vi "CreatePrivateEvents.vi"(8 "error in (no error)":errorcluster, 11 "Lockin.DAQ":refnum<class "Instrument.DAQ.lvclass">) -> (0 "error out":errorcluster, 3 "Lockin.DAQ out":refnum<class "Instrument.DAQ.lvclass">)   [LabVIEW 2019, in "Instrument.Lockin.lvlib" / "Instrument.DAQ.lvclass"]
doc: "---------------------------------------------------------------\nJKI State Machine Objects™\nhttp://jki.net/state-machine-objects/\nCopyright (C) 2005-2015, JKI <info@jki.net>\nALL RIGHTS RESERVEDJKI State Machine Objects (SMO) 1.0.0.4\nJKI - JKI\nCopyright (c) 2015, JKI"
uses:
  Instrument.DAQ.lvclass
  Typedefs/PrivateEvents--DAQ.setAOconfig.ctl
  Typedefs/DAQ.Config.AO--Cluster--Array.ctl
  Typedefs/DAQ.Config.AO.Range--enum.ctl
  Typedefs/DAQ.TerminalConfiguration--ring.ctl
  Typedefs/DAQ.Type--enum.ctl
  Typedefs/PrivateEvents--DAQ.setAIconfig.ctl
  Typedefs/DAQ.Config.AI--Cluster--Array.ctl
  Typedefs/DAQ.Config.AI.Coupling--enum.ctl
  Typedefs/DAQ.Config.AI.Range--enum.ctl
  DAQmx/typedefs/Simulation Mode--enum.ctl
  Typedefs/PrivateEvents--DAQ.setAO.ctl
  Typedefs/AO.Channel--Cluster--Array.ctl
  Typedefs/AO.Channel--Cluster.ctl
  Typedefs/AO.Channel.Function--Enum.ctl
  Typedefs/PrivateEvents--DAQ.setREF.ctl
  Typedefs/REF.Channel--Cluster--Array.ctl
  Typedefs/REF.Channel--Cluster.ctl
  Typedefs/PrivateEvents--DAQ.setSampling.ctl
  Typedefs/DAQ.Sampling--Cluster.ctl
  Typedefs/DAQ.Sampling.Sampling--Cluster.ctl
  Typedefs/PrivateEvents--DAQ.setState.ctl
  Typedefs/State--enum.ctl
  Typedefs/PrivateEvents--DAQ.setInputGain.ctl
  Typedefs/PrivateEvents--DAQ.setSweep.ctl
  Typedefs/Sweep.Configuration--Cluster.ctl
  Typedefs/Sweep.Channel--Cluster--Array.ctl
  Typedefs/Sweep.Channel--Cluster.ctl
  Typedefs/Sweep.Pattern--Enum.ctl
  Typedefs/PrivateEvents--DAQ.measureOffset.ctl
  Typedefs/PrivateEvents--DAQ.zeroOffset.ctl
  Typedefs/PrivateEvents--DAQ.setPreFilter.ctl
  Typedefs/Configuration.Prefilter--Cluster.ctl
  Typedefs/PrivateEvents--DAQ.autoConfigureDAQ.ctl
  Typedefs/PrivateEvents--DAQ.setCalibration.ctl
  Typedefs/PrivateEvents--DAQ.setOutputGain.ctl
  Typedefs/PrivateEvents--DAQ.setAI.ctl
  Typedefs/AI.Channel--Cluster--Array.ctl
  Typedefs/AI.Channel--Cluster.ctl
  Typedefs/PrivateEvents--DAQ.zeroPhase.ctl
  Typedefs/PrivateEvents--DAQ.setAmplitudeLimit.ctl
  Typedefs/Configuration.AmplitudeLimit--Cluster.ctl
  Typedefs/PrivateEvents--DAQ.setLinkFrequencies.ctl
  Typedefs/Configuration.LinkFrequencies--Cluster.ctl
  Typedefs/PrivateEvents--DAQ.showUI.ctl
  Typedefs/PrivateEvents--DAQ.setInputOffset.ctl
  Typedefs/PrivateEvents--DAQ.setDCLimit.ctl
  Typedefs/Configuration.DCLimit--Cluster.ctl
  Typedefs/PrivateEvents--DAQ.setDutyCycle.ctl
  Typedefs/Configuration.DutyCycle--Cluster.ctl
  Instrument.DAQ.lvclass/Instrument.DAQ.ctl
  <vilib>/JKI/JKI SMO/SMO/SMO.lvclass
  DAQmx/DAQmx.lvclass
panel:
  # "For instructions on how to use the JKI State Machine Objects, examples and video tutorials, visit:\nhttp://jki.net/state-machine-objects/\n\nJKI State Machine Objects™\nhttp://jki.net/state-machine-objects/\nCopyright (C) 2005-2015, JKI <info@jki.net>\nALL RIGHTS RESERVED"
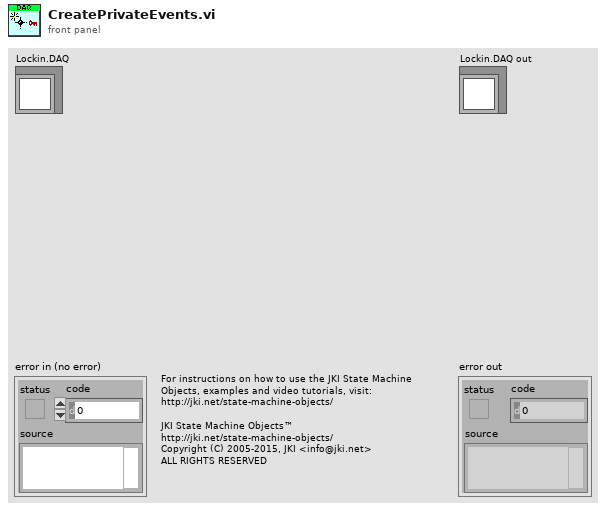
[diagram p1: front panel]
types:
  T1 = typedef "Instrument.Lockin.lvlib/Instrument.DAQ.lvclass/PrivateEvents--DAQ.setDutyCycle.ctl" = cluster{"Duty Cycle":T2}
  T2 = typedef "Instrument.Lockin.lvlib/Instrument.DAQ.lvclass/Configuration.DutyCycle--Cluster.ctl" = cluster{"Option?":bool, "Duty Cycle (%)":dbl}
  T3 = typedef "Instrument.Lockin.lvlib/Instrument.DAQ.lvclass/PrivateEvents--DAQ.setDCLimit.ctl" = cluster{"DC Limit":T4}
  T4 = typedef "Instrument.Lockin.lvlib/Instrument.DAQ.lvclass/Configuration.DCLimit--Cluster.ctl" = cluster{"Limit (V)":dbl}
  T5 = typedef "Instrument.Lockin.lvlib/Instrument.DAQ.lvclass/PrivateEvents--DAQ.setInputOffset.ctl" = cluster{"Input Offset":dbl[]}
  T6 = typedef "Instrument.Lockin.lvlib/Instrument.DAQ.lvclass/PrivateEvents--DAQ.showUI.ctl" = bool
  T7 = typedef "Instrument.Lockin.lvlib/Instrument.DAQ.lvclass/PrivateEvents--DAQ.setLinkFrequencies.ctl" = cluster{"Link Frequencies":T8}
  T8 = typedef "Instrument.Lockin.lvlib/Instrument.DAQ.lvclass/Configuration.LinkFrequencies--Cluster.ctl" = cluster{"Link?":bool, "Frequency (Hz)":dbl}
  T9 = typedef "Instrument.Lockin.lvlib/Instrument.DAQ.lvclass/PrivateEvents--DAQ.setAmplitudeLimit.ctl" = cluster{"Amplitude Limit ":T10}
  T10 = typedef "Instrument.Lockin.lvlib/Instrument.DAQ.lvclass/Configuration.AmplitudeLimit--Cluster.ctl" = cluster{"Limit (V)":dbl}
  T11 = typedef "Instrument.Lockin.lvlib/Instrument.DAQ.lvclass/PrivateEvents--DAQ.zeroPhase.ctl" = bool
  T12 = typedef "Instrument.Lockin.lvlib/Instrument.DAQ.lvclass/PrivateEvents--DAQ.setAI.ctl" = cluster{"AI Channels":T13}
  T13 = typedef "Instrument.Lockin.lvlib/Instrument.DAQ.lvclass/AI.Channel--Cluster--Array.ctl" = T14[]
  T14 = typedef "Instrument.Lockin.lvlib/Instrument.DAQ.lvclass/AI.Channel--Cluster.ctl" = cluster{"Enable?":bool, "Channel":i32, "References":u16[], "reference index":i32}
  T15 = typedef "Instrument.Lockin.lvlib/Instrument.DAQ.lvclass/PrivateEvents--DAQ.setOutputGain.ctl" = cluster{"Output Gain":dbl[]}
  T16 = typedef "Instrument.Lockin.lvlib/Instrument.DAQ.lvclass/PrivateEvents--DAQ.setCalibration.ctl" = enum16{"Check", "Calibrate"}
  T17 = typedef "Instrument.Lockin.lvlib/Instrument.DAQ.lvclass/PrivateEvents--DAQ.autoConfigureDAQ.ctl" = bool
  T18 = typedef "Instrument.Lockin.lvlib/Instrument.DAQ.lvclass/PrivateEvents--DAQ.setPreFilter.ctl" = cluster{"PreFilter":T19}
  T19 = typedef "Instrument.Lockin.lvlib/Instrument.DAQ.lvclass/Configuration.Prefilter--Cluster.ctl" = cluster{"60 Hz":bool, "Low Pass":bool, "Low Pass Cutoff (Hz)":dbl}
  T20 = typedef "Instrument.Lockin.lvlib/Instrument.DAQ.lvclass/PrivateEvents--DAQ.zeroOffset.ctl" = bool
  T21 = typedef "Instrument.Lockin.lvlib/Instrument.DAQ.lvclass/PrivateEvents--DAQ.measureOffset.ctl" = bool
  T22 = typedef "Instrument.Lockin.lvlib/Instrument.DAQ.lvclass/PrivateEvents--DAQ.setSweep.ctl" = cluster{"setSweep":T23}
  T23 = typedef "Instrument.Lockin.lvlib/Instrument.DAQ.lvclass/Sweep.Configuration--Cluster.ctl" = cluster{"sweepTime":dbl, "initialWaitTime":dbl, "returnToStart":bool, "sweepChannels":T24}
  T24 = typedef "Instrument.Lockin.lvlib/Instrument.DAQ.lvclass/Sweep.Channel--Cluster--Array.ctl" = T25[]
  T25 = typedef "Instrument.Lockin.lvlib/Instrument.DAQ.lvclass/Sweep.Channel--Cluster.ctl" = cluster{"Enable?":bool, "Channel":u16, "Start":dbl, "End":dbl, "Pattern":T26, "Table":dbl[]}
  T26 = typedef "Instrument.Lockin.lvlib/Instrument.DAQ.lvclass/Sweep.Pattern--Enum.ctl" = enum16{"Ramp /", "Ramp /\\", "Smooth Ramp _/", "Smooth Ramp _/\\_", "Table"}
  T27 = typedef "Instrument.Lockin.lvlib/Instrument.DAQ.lvclass/PrivateEvents--DAQ.setInputGain.ctl" = cluster{"Input Gain":dbl[]}
  T28 = typedef "Instrument.Lockin.lvlib/Instrument.DAQ.lvclass/PrivateEvents--DAQ.setState.ctl" = cluster{"setState":T29}
  T29 = typedef "Instrument.Lockin.lvlib/Instrument.DAQ.lvclass/State--enum.ctl" = enum16{"start", "stop", "reset", "start sweep", "stop sweep"}
  T30 = typedef "Instrument.Lockin.lvlib/Instrument.DAQ.lvclass/PrivateEvents--DAQ.setSampling.ctl" = cluster{"Sampling":T31}
  T31 = typedef "Instrument.Lockin.lvlib/Instrument.DAQ.lvclass/DAQ.Sampling--Cluster.ctl" = cluster{"Sampling":T32, "Fs_Out":dbl}
  T32 = typedef "Instrument.Lockin.lvlib/Instrument.DAQ.lvclass/DAQ.Sampling.Sampling--Cluster.ctl" = cluster{"Fs":dbl, "#s":i32}
  T33 = typedef "Instrument.Lockin.lvlib/Instrument.DAQ.lvclass/PrivateEvents--DAQ.setREF.ctl" = cluster{"REF Channels":T34}
  T34 = typedef "Instrument.Lockin.lvlib/Instrument.DAQ.lvclass/REF.Channel--Cluster--Array.ctl" = T35[]
  T35 = typedef "Instrument.Lockin.lvlib/Instrument.DAQ.lvclass/REF.Channel--Cluster.ctl" = cluster{"Enable?":bool, "Channel":i32, "Frequency":dbl, "Phase":dbl, "TC":dbl, "Roll-Off":i32}
  T36 = typedef "Instrument.Lockin.lvlib/Instrument.DAQ.lvclass/PrivateEvents--DAQ.setAO.ctl" = cluster{"AO Channels":T37}
  T37 = typedef "Instrument.Lockin.lvlib/Instrument.DAQ.lvclass/AO.Channel--Cluster--Array.ctl" = T38[]
  T38 = typedef "Instrument.Lockin.lvlib/Instrument.DAQ.lvclass/AO.Channel--Cluster.ctl" = cluster{"Enable?":bool, "Channel":i32, "Amplitude":dbl, "Offset":dbl, "Frequency":dbl, "Phase":dbl, "Function":T39, "Sweeping?":bool, "Limit AC":bool, "Limit DC?":bool, "Duty Cycle":bool}
  T39 = typedef "Instrument.Lockin.lvlib/Instrument.DAQ.lvclass/AO.Channel.Function--Enum.ctl" = enum16{"sine", "square", "triangle", "saw"}
  T40 = typedef "Instrument.Lockin.lvlib/Instrument.DAQ.lvclass/PrivateEvents--DAQ.setAIconfig.ctl" = cluster{"AI Configuration":T41, "Simulation mode":T46}
  T41 = typedef "Instrument.Lockin.lvlib/Instrument.DAQ.lvclass/DAQ.Config.AI--Cluster--Array.ctl" = cluster{"Channels":tag, "Coupling":T42, "Range":T43, "terminal configuration":T44, "Type":T45}[]
  T42 = typedef "Instrument.Lockin.lvlib/Instrument.DAQ.lvclass/DAQ.Config.AI.Coupling--enum.ctl" = u16
  T43 = typedef "Instrument.Lockin.lvlib/Instrument.DAQ.lvclass/DAQ.Config.AI.Range--enum.ctl" = enum16{"±0.316", "±1.00", "±3.16", "±10.0", "±31.6", "±42.4", ""}
  T44 = typedef "Instrument.Lockin.lvlib/Instrument.DAQ.lvclass/DAQ.TerminalConfiguration--ring.ctl" = i32
  T45 = typedef "Instrument.Lockin.lvlib/Instrument.DAQ.lvclass/DAQ.Type--enum.ctl" = enum16{"None", "USB-4431", "PXI-446x"}
  T46 = typedef "DAQmx.lvclass/Simulation Mode--enum.ctl" = enum16{"AI = HW simulated", "AI = noise*AO", "AI = waveguide"}
  T47 = typedef "Instrument.Lockin.lvlib/Instrument.DAQ.lvclass/PrivateEvents--DAQ.setAOconfig.ctl" = cluster{"AO Configuration":T48}
  T48 = typedef "Instrument.Lockin.lvlib/Instrument.DAQ.lvclass/DAQ.Config.AO--Cluster--Array.ctl" = cluster{"Channels":tag, "Range":T49, "terminal configuration":T44, "Type":T45}[]
  T49 = typedef "Instrument.Lockin.lvlib/Instrument.DAQ.lvclass/DAQ.Config.AO.Range--enum.ctl" = enum16{"±0.1", "±1.0", "±3.5", "±10.0", ""}
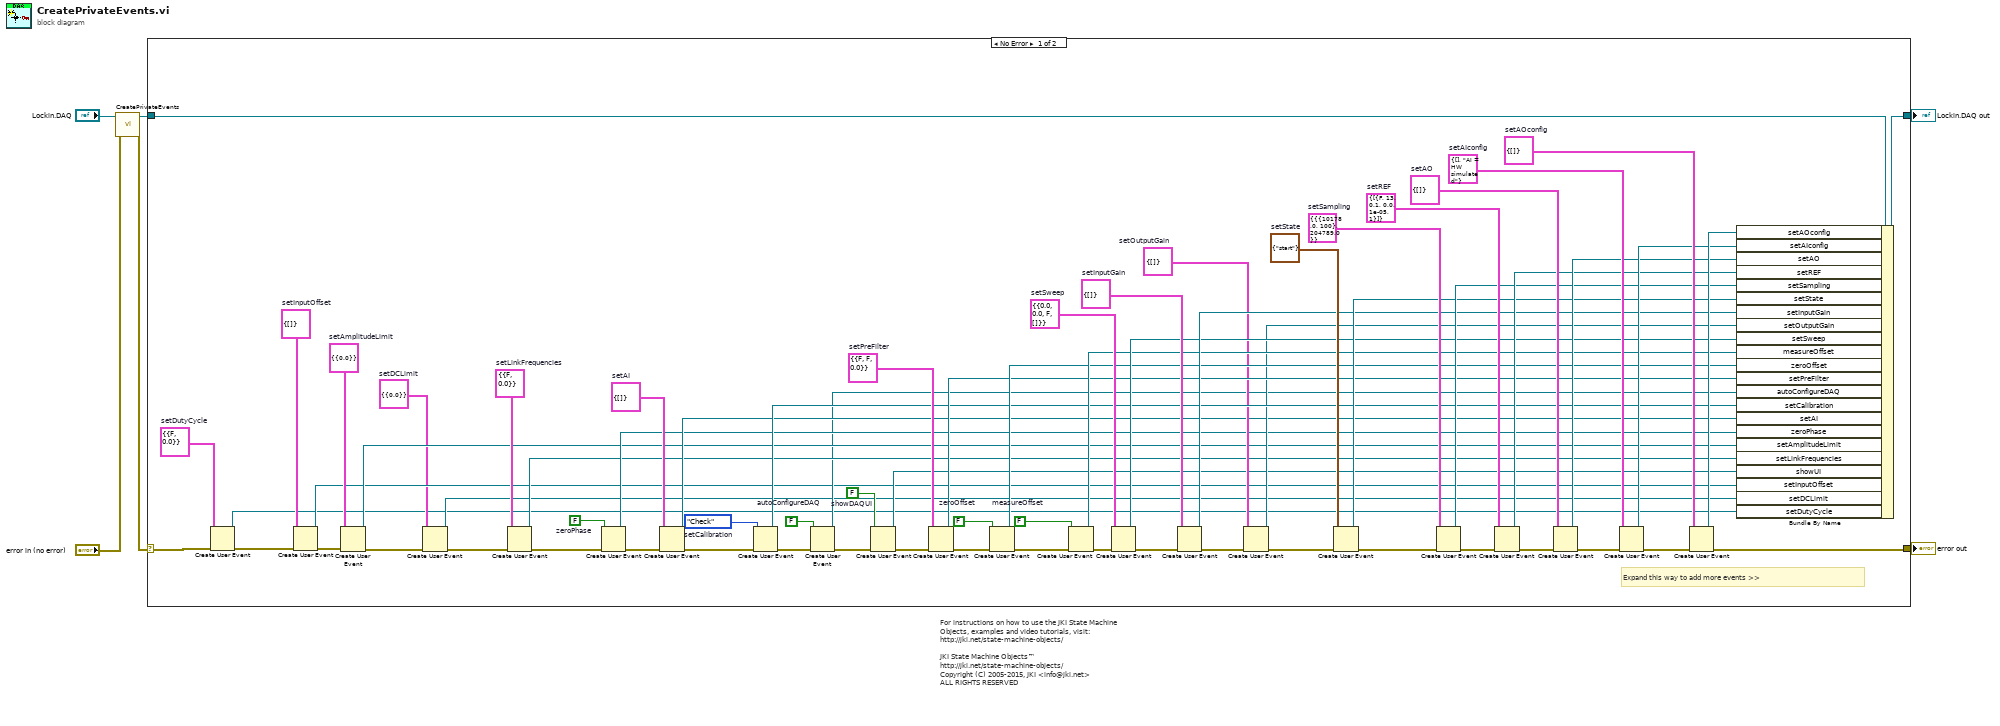
[diagram p0: block diagram]
diagram:
  # "For instructions on how to use the JKI State Machine Objects, examples and video tutorials, visit:\nhttp://jki.net/state-machine-objects/\n\nJKI State Machine Objects™\nhttp://jki.net/state-machine-objects/\nCopyright (C) 2005-2015, JKI <info@jki.net>\nALL RIGHTS RESERVED"
  n1 = call-parent "CreatePrivateEvents.vi"("error in (no error)"="error in (no error)", "SMO"="Lockin.DAQ") -> ("error out"=w1:errorcluster, "SMO out"=w3:refnum<class "Instrument.DAQ.lvclass">)  [unwired: 8 in]
  n2 = case shown="No Error" w1 {
    selector: w1 -> [w9 w77]
    tunnel: [w73 w77] -> w5
    tunnel: [w74 w76] -> w6
    tunnel: w3 -> [w75 w76]
    frame No Error {
      w10 = T1 {"Duty Cycle"={"Option?"=FALSE, "Duty Cycle (%)"=0.0}}  # setDutyCycle
      w14 = T3 {"DC Limit"={"Limit (V)"=0.0}}  # setDCLimit
      w17 = T5 {"Input Offset"=[]}  # setInputOffset
      w21 = T6 FALSE  # showDAQUI
      w25 = T7 {"Link Frequencies"={"Link?"=FALSE, "Frequency (Hz)"=0.0}}  # setLinkFrequencies
      w26 = T9 {"Amplitude Limit "={"Limit (V)"=0.0}}  # setAmplitudeLimit
      w29 = T11 FALSE  # zeroPhase
      w32 = T12 {"AI Channels"=[]}  # setAI
      w35 = T15 {"Output Gain"=[]}  # setOutputGain
      w39 = PrivateEvents--DAQ.setCalibration."Check"  # setCalibration
      w41 = T17 FALSE  # autoConfigureDAQ
      w43 = T18 {"PreFilter"={"60 Hz"=FALSE, "Low Pass"=FALSE, "Low Pass Cutoff (Hz)"=0.0}}  # setPreFilter
      w46 = T20 FALSE  # zeroOffset
      w49 = T21 FALSE  # measureOffset
      w52 = T22 {"setSweep"={"sweepTime"=0.0, "initialWaitTime"=0.0, "returnToStart"=FALSE, "sweepChannels"=[]}}  # setSweep
      w55 = T27 {"Input Gain"=[]}  # setInputGain
      w57 = T28 {"setState"=enum."start"}  # setState
      w60 = T30 {"Sampling"={"Sampling"={"Fs"=10178.0, "#s"=100}, "Fs_Out"=204789.0}}  # setSampling
      w63 = T33 {"REF Channels"=[{"Enable?"=FALSE, "Channel"=13, "Frequency"=0.1, "Phase"=0.0, "TC"=1e-05, "Roll-Off"=1}]}  # setREF
      w66 = T36 {"AO Channels"=[]}  # setAO
      w69 = T40 {"AI Configuration"=[], "Simulation mode"=enum."AI = HW simulated"}  # setAIconfig
      w72 = T47 {"AO Configuration"=[]}  # setAOconfig
      # "Expand this way to add more events >>"
      n3 = Create User Event(user event datatype=w10, error in=w9) -> (user event=w7:refnum<user-event>, error out=w8:errorcluster)
      n4 = Create User Event(user event datatype=w17, error in=w8) -> (user event=w15:refnum<user-event>, error out=w16:errorcluster)
      n5 = Create User Event(user event datatype=w26, error in=w16) -> (user event=w24:refnum<user-event>, error out=w13:errorcluster)
      n6 = Create User Event(user event datatype=w14, error in=w13) -> (user event=w11:refnum<user-event>, error out=w12:errorcluster)
      n7 = Create User Event(user event datatype=w25, error in=w12) -> (user event=w23:refnum<user-event>, error out=w27:errorcluster)
      n8 = Create User Event(user event datatype=w29, error in=w27) -> (user event=w28:refnum<user-event>, error out=w30:errorcluster)
      n9 = Create User Event(user event datatype=w32, error in=w30) -> (user event=w31:refnum<user-event>, error out=w33:errorcluster)
      n10 = Create User Event(user event datatype=w39, error in=w33) -> (user event=w38:refnum<user-event>, error out=w40:errorcluster)
      n11 = Create User Event(user event datatype=w41, error in=w40) -> (user event=w22:refnum<user-event>, error out=w20:errorcluster)
      n12 = Create User Event(user event datatype=w21, error in=w20) -> (user event=w19:refnum<user-event>, error out=w18:errorcluster)
      n13 = Create User Event(user event datatype=w43, error in=w18) -> (user event=w42:refnum<user-event>, error out=w44:errorcluster)
      n14 = Create User Event(user event datatype=w46, error in=w44) -> (user event=w45:refnum<user-event>, error out=w47:errorcluster)
      n15 = Create User Event(user event datatype=w49, error in=w47) -> (user event=w48:refnum<user-event>, error out=w50:errorcluster)
      n16 = Create User Event(user event datatype=w52, error in=w50) -> (user event=w51:refnum<user-event>, error out=w53:errorcluster)
      n17 = Create User Event(user event datatype=w55, error in=w53) -> (user event=w54:refnum<user-event>, error out=w37:errorcluster)
      n18 = Create User Event(user event datatype=w35, error in=w37) -> (user event=w34:refnum<user-event>, error out=w36:errorcluster)
      n19 = Create User Event(user event datatype=w57, error in=w36) -> (user event=w56:refnum<user-event>, error out=w58:errorcluster)
      n20 = Create User Event(user event datatype=w60, error in=w58) -> (user event=w59:refnum<user-event>, error out=w61:errorcluster)
      n21 = Create User Event(user event datatype=w63, error in=w61) -> (user event=w62:refnum<user-event>, error out=w64:errorcluster)
      n22 = Create User Event(user event datatype=w66, error in=w64) -> (user event=w65:refnum<user-event>, error out=w67:errorcluster)
      n23 = Create User Event(user event datatype=w69, error in=w67) -> (user event=w68:refnum<user-event>, error out=w70:errorcluster)
      n24 = Create User Event(user event datatype=w72, error in=w70) -> (user event=w71:refnum<user-event>, error out=w73:errorcluster)
      n25 = Bundle By Name(cluster=w75, "setAOconfig"=w71, "setAIconfig"=w68, "setAO"=w65, "setREF"=w62, "setSampling"=w59, "setState"=w56, "setInputGain"=w54, "setOutputGain"=w34, "setSweep"=w51, "measureOffset"=w48, "zeroOffset"=w45, "setPreFilter"=w42, "autoConfigureDAQ"=w22, "setCalibration"=w38, "setAI"=w31, "zeroPhase"=w28, "setAmplitudeLimit"=w24, "setLinkFrequencies"=w23, "showUI"=w19, "setInputOffset"=w15, "setDCLimit"=w11, "setDutyCycle"=w7) -> (w74:refnum<class "Instrument.DAQ.lvclass">)
    }
    frame Error {
    }
  }
  "error out" <- w5
  "Lockin.DAQ out" <- w6
